vi "AIT 429 - Add Channels.vi"(8 "error in (no error)":errorcluster, 11 "Node Ptr":u64 format="%.0x") -> (0 "error out":errorcluster)   [LabVIEW 2011, in "AIT 429 Custom Device.lvlib"]
uses:
  AIT 429 Custom Device.lvlib
  Controls/Channel Setup.ctl
  Controls and Global/Start Bit.ctl
  Controls and Global/Number of Bits.ctl
  <vilib>/NI Veristand/Custom Device API/Custom Device Channel Type.ctl
  <vilib>/NI Veristand/Custom Device API/Custom Device Channel.ctl
  Controls and Global/Global.vi
  <vilib>/NI Veristand/Custom Device API/Get Item Property (U32).vi
  <vilib>/NI Veristand/Custom Device API/Custom Device API.lvlib
panel:
  in  "Cancel":bool
  in  "OK":bool
  in  "Parameters to add":T1[](array[typedef]) {"Number of Bits" min=1 max=32}
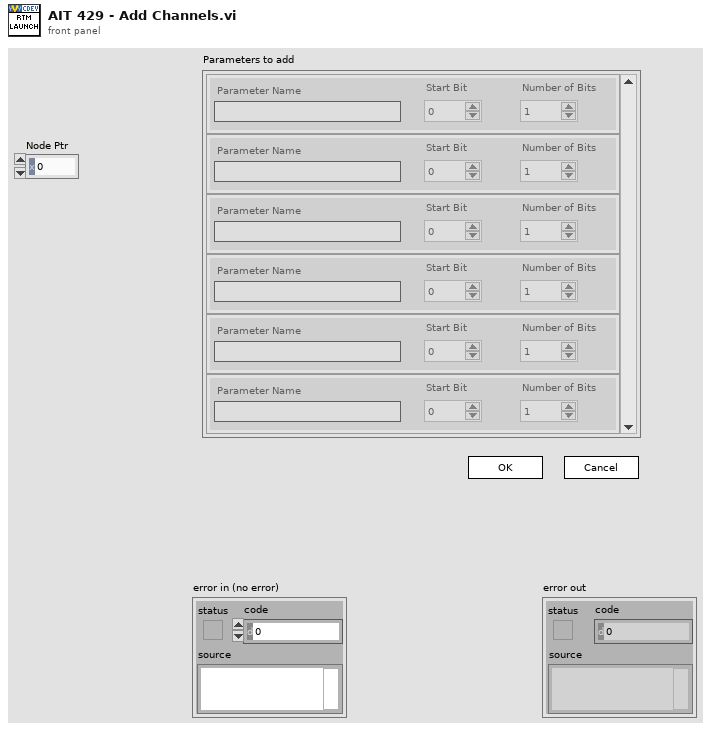
[diagram p1: front panel]
types:
  T1 = typedef "AIT 429 Custom Device.lvlib/Channel Setup.ctl" = cluster{"Parameter Name":string, "Start Bit":T2, "Number of Bits":T3}
  T2 = typedef "AIT 429 Custom Device.lvlib/Start Bit.ctl" = i32
  T3 = typedef "AIT 429 Custom Device.lvlib/Number of Bits.ctl" = i32
  T4 = typedef "Custom Device API.lvlib/Custom Device Channel Type.ctl" = enum16{"Input", "Output"}
  T5 = typedef "Custom Device API.lvlib/Custom Device Channel.ctl" = cluster{"Type":T4, "Units":string, "Default Value":dbl, "Faultable":bool, "Scalable":bool}
  T6 = typedef "Custom Device API.lvlib/Custom Device Item Ref.ctl" = u64
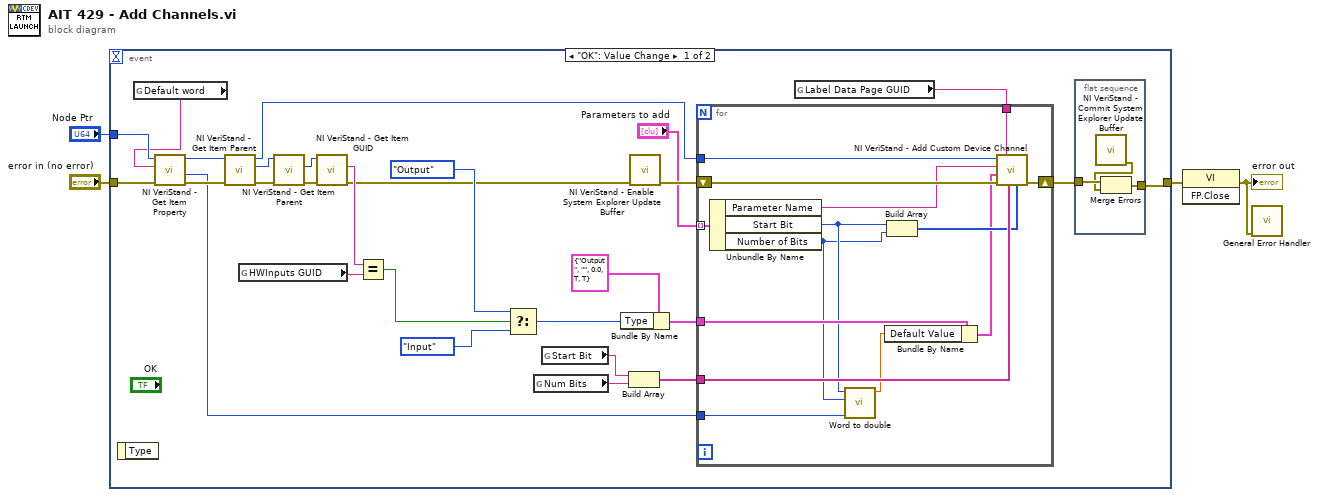
[diagram p0: block diagram]
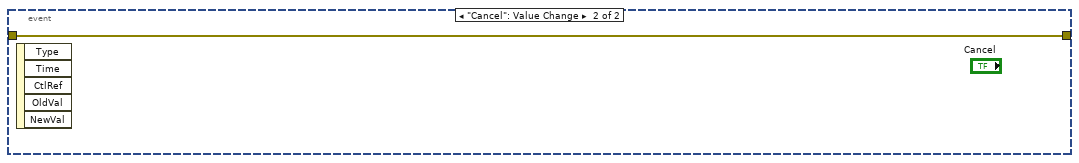
[diagram p2: hidden frame]
diagram:
  n1 = event shown="[0] \"OK\": Value Change" {
    selector: _ -> [_ _]
    dyn-events: _ -> [_ _]
    timeout: _ -> [_ _]
    tunnel: [w6 w50] -> w2
    tunnel: "error in (no error)" -> [w11 w50]
    tunnel: "Node Ptr" -> [w10 _]
    event "OK": Value Change {
      n2 = event-data() -> ()  [unwired: 1 in, 1 out]
      n3 = global read "Global.vi" "Default word"() -> (w9:string)
      n4 = call-poly <vilib>:"NI VeriStand - Get Item Property.vi"("error in (no error)"=w11, "Property Name"=w9, "Item Ref in"=w10) -> ("error out"=w13:errorcluster, "Value"=w8:u32, "Item Ref out"=w12:T6)  [unwired: 5 in, 1 out]
      n5 = call <vilib>:"NI VeriStand - Get Item Parent.vi"("error in (no error)"=w13, "Item Ref in"=w12) -> ("error out"=w29:errorcluster, "Parent Ref"=w26:T6, "Item Ref out"=w18:T6)  [unwired: 6 in, 1 out]
      n6 = global read "Global.vi" "HWInputs GUID"() -> (w20:string)
      n7 = call <vilib>:"NI VeriStand - Get Item Parent.vi"("error in (no error)"=w29, "Item Ref in"=w26) -> ("error out"=w28:errorcluster, "Parent Ref"=w27:T6)  [unwired: 6 in, 2 out]
      n8 = call <vilib>:"NI VeriStand - Get Item GUID.vi"("error in (no error)"=w28, "Item Ref in"=w27) -> ("error out"=w5:errorcluster, "GUID"=w19:string)  [unwired: 7 in, 1 out]
      n9 = Equal?(x=w19, y=w20) -> (x = y?=w14:bool)
      n10 = Select(t=Custom_Device_Channel_Type."Output" ("Type"), s=w14, f=Custom_Device_Channel_Type."Input" ("Type")) -> (s? t:f=w23:T4)
      n11 = global read "Global.vi" "Num Bits"() -> (w31:string)
      n12 = global read "Global.vi" "Start Bit"() -> (w16:string)
      n13 = Bundle By Name(cluster=T5 {"Type"=enum."Output", "Units"="", "Default Value"=0.0, "Faultable"=TRUE, "Scalable"=TRUE} ("Channel"), "Type"=w23) -> (w25:T5)
      n14 = Build Array(w16, w31) -> (w17:string[])
      n15 = call <vilib>:"NI VeriStand - Enable System Explorer Update Buffer.vi"("error in (no error)"=w5) -> ("error out"=w32:errorcluster)  [unwired: 10 in]
      n16 = global read "Global.vi" "Label Data Page GUID"() -> (w30:string)
      n17 = for {
        shift-right: [w48] -> w7
        shift-left: w32 -> [w49]
        tunnel: w18 -> [w46]
        tunnel: w17 -> [w47]
        tunnel: w25 -> [w41]
        tunnel: w30 -> [w45]
        tunnel: "Parameters to add" -> [w44] mode=indexing
        tunnel: w8 -> [w39]
        n18 = Unbundle By Name(w44) -> ("Parameter Name"=w43:string, "Start Bit"=w37:T2, "Number of Bits"=w36:T3)
        n19 = call "Word to double.vi"("word"=w39, "Number of Bits"=w36, "Start Bit"=w37) -> ("Double"=w38:dbl)  [unwired: 8 in]
        n20 = Bundle By Name(cluster=w41, "Default Value"=w38) -> (w40:T5)
        n21 = Build Array(w37, w36) -> (w42:T3[])
        n22 = call <vilib>:"NI VeriStand - Add Custom Device Channel.vi"("Property Values"=w42, "Property names"=w47, "GUID (Default Channel)"=w45, "error in (no error)"=w49, "Channel"=w40, "Channel Name"=w43, "Parent Ref in"=w46) -> ("error out"=w48:errorcluster)  [unwired: 1 in, 3 out]
      }
      n23 = flat-sequence {
        tunnel: w7 -> [w35]
        tunnel: [w33] -> w6
        frame #0 {
          n24 = call <vilib>:"NI VeriStand - Commit System Explorer Update Buffer.vi"() -> ("error out"=w34:errorcluster)  [unwired: 11 in]
          n25 = Merge Errors(w35, w34) -> (w33:errorcluster)
        }
      }
    }
    event "Cancel": Value Change {
      n26 = event-data() -> ()  [unwired: 1 in, 5 out]
    }
  }
  n27 = invoke class="VI" method="FP.Close"(error in=w2) -> (error out=w1:errorcluster)  [unwired: 2 in, 2 out]
  "error out" <- w1
  n28 = call <vilib>:"General Error Handler.vi"("error in (no error)"=w1) -> ()  [unwired: 10 in, 5 out]
